vi "Configure Bar Graph (IO).vi"(0 "VISA resource name":refnum<visa-resource-name>, 5 "Channel (0001)":string="0001", 7 "Base Position (0: Lower)":u16(ring) items=["Lower", "Center", "Upper"], 9 "Division (10)":i32=10 min=4 max=12, 11 "error in (no error)":errorcluster) -> (4 "VISA resource name out":refnum<visa-resource-name>, 6 "Channel":string, 15 "error out":errorcluster)   [LabVIEW 2020, in "Yokogawa GX Series.lvlib"]
doc: "Sets the bar graph display of an I/O channel.\n\nCommand: SBarIO"
uses:
  <instrlib>/Yokogawa GX Series/Yokogawa GX Series.lvlib
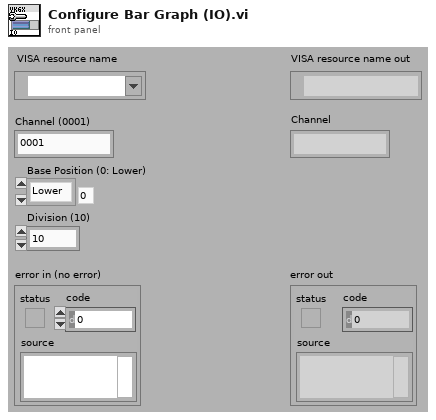
[diagram p1: front panel]
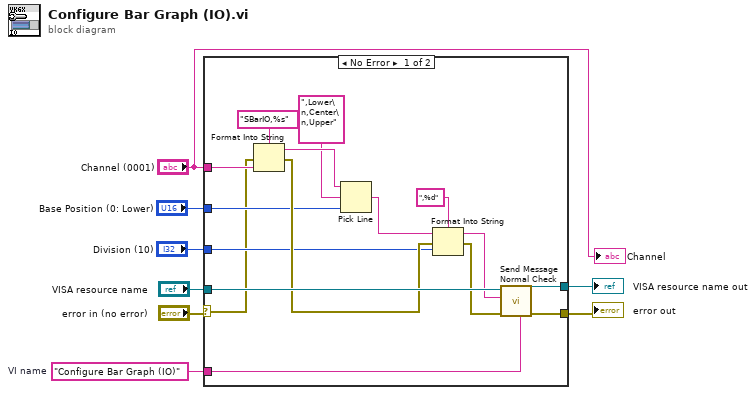
[diagram p0: block diagram]
diagram:
  w7 = "Configure Bar Graph (IO)"  # VI name
  n1 = case shown="No Error" "error in (no error)" {
    selector: "error in (no error)" -> [w9 w25]
    tunnel: "VISA resource name" -> [w24 w26]
    tunnel: w7 -> [w23 _]
    tunnel: [w22 w26] -> w6
    tunnel: [w21 w25] -> w5
    tunnel: "Division (10)" -> [w17 _]
    tunnel: "Base Position (0: Lower)" -> [w14 _]
    tunnel: "Channel (0001)" -> [w10 _]
    frame No Error {
      n2 = Format Into String(format string="SBarIO,%s", error in=w9, w10) -> (resulting string=w13:string, error out=w18:errorcluster)  [unwired: 1 in]
      n3 = Pick Line(string ("")=w13, multi-line string=",Lower\n,Center\n,Upper", line index=w14) -> (output string=w11:string)
      n4 = Format Into String(format string=",%d", initial string=w11, error in=w18, w17) -> (resulting string=w16:string, error out=w15:errorcluster)
      n5 = call <instrlib>:"Send Message Normal Check.vi"("Source (\"\")"=w23, "error in (no error)"=w15, "Send Message (\"\")"=w16, "VISA resource name"=w24) -> ("error out"=w21:errorcluster, "VISA resource name out"=w22:refnum<visa-resource-name>)  [unwired: 2 in, 4 out]
    }
    frame Error {
    }
  }
  "error out" <- w5
  "VISA resource name out" <- w6
  "Channel" <- "Channel (0001)"
